vi "Robot Main.vi"   [LabVIEW 2013]
doc: "This VI imlements the framework and scheduler for your robotics program. It should not be necessary to modify the framework. You are expected to add your code to the VIs called from Robot Main, the ones located in the Team Code within the project."
panel:
  # "2014 Vision Practice"
  # "Version 0.1"
  # "Todo"
  # "Controls"
  # "PWM"
  # "DIO"
  # "Relay"
  # "Analog"
  # "Solenoid"
  # "JS 1\nX Axis: Arcade Drive\nY Axis: Arcade Drive\nZ Axis:\nButton 1: GoTo Shoot Location\nButton 2: Toggle Vision\nButton 3: To Driver Control\nButton 4:\nButton 5:\nButton 6: \nButton 7: \nButton 8: \nButton 9: \nButton 10:\nButton 11: \nButton 12:"
  # "JS 2\nX Axis: \nY Axis: \nZ Axis: \nButton 1:  \nButton 2:  \nButton 3: \nButton 4: \nButton 5: \nButton 6: \nButton 7:  \nButton 8: \nButton 9: \nButton 10: \nButton 11:  \nButton 12:"
  # "1 a): \n1 b): \n2 a): \n2 b): \n3 a): \n3 b): \n     4: \n     5: \n     6: \n     7: \n     8: \n     9: \n   10:"
  # "1: \n  2: \n  3: \n  4: \n  5: \n  6: \n  7: \n  8: \n  9: \n10:\n11:\n12:\n13: \n14: Pneumatic Pressure Switch"
  # "1: \n2:\n3:\n4:\n5:\n6:\n7:\n8:"
  # "1:\n2:\n3:\n4:\n5:\n6:\n7:\n8:"
  # "1: Shifter A \n2: Shifter B\n3: \n4: \n5: \n6: \n7:\n8:"
  # "JS 3\nX Axis: \nY Axis: \nZ Axis: \nButton 1: \nButton 2: \nButton 3: \nButton 4: \nButton 5:\nButton 6: \nButton 7: \nButton 8: \nButton 9: \nButton 10: \nButton 11: \nButton 12:"
  # "- Vision"
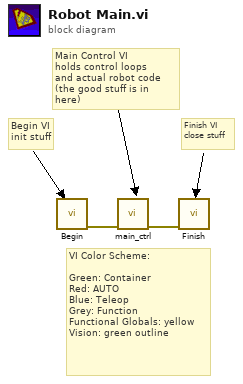
[diagram p0: block diagram]
diagram:
  # "Finish VI\nclose stuff"
  # "Main Control VI\nholds control loops\nand actual robot code\n(the good stuff is in here)"
  # "Begin VI\ninit stuff"
  # "VI Color Scheme:\n\nGreen: Container\nRed: AUTO\nBlue: Teleop\nGrey: Function\nFunctional Globals: yellow\nVision: green outline"
  n1 = call "Begin.vi"() -> ("error out"=w2:errorcluster)  [unwired: 1 in, 10 out]
  n2 = call "main_ctrl.vi"("error in"=w2) -> ("error out"=w1:errorcluster)  [unwired: 10 in]
  n3 = call "Finish.vi"("error in"=w1) -> ()  [unwired: 7 in]
